vi "test.vi"() -> ()   [LabVIEW 2017]
uses:
  Global/Global 1.vi
panel:
  in  "send":bool
  in  "stop":bool
  in  "scan 6":string
  in  "scan 5":string
  in  "scan 4":string
  in  "scan 3":string
  in  "scan 2":string
  in  "scan 1":string
  in  "cycle start 6":bool
  in  "cycle start 5":bool
  in  "cycle start 4":bool
  in  "cycle start 3":bool
  in  "cycle start 2":bool
  in  "result  6":bool
  in  "cycle start 1":bool
  in  "result  5":bool
  in  "result  4":bool
  in  "result  3":bool
  in  "result  2":bool
  in  "result 1":bool
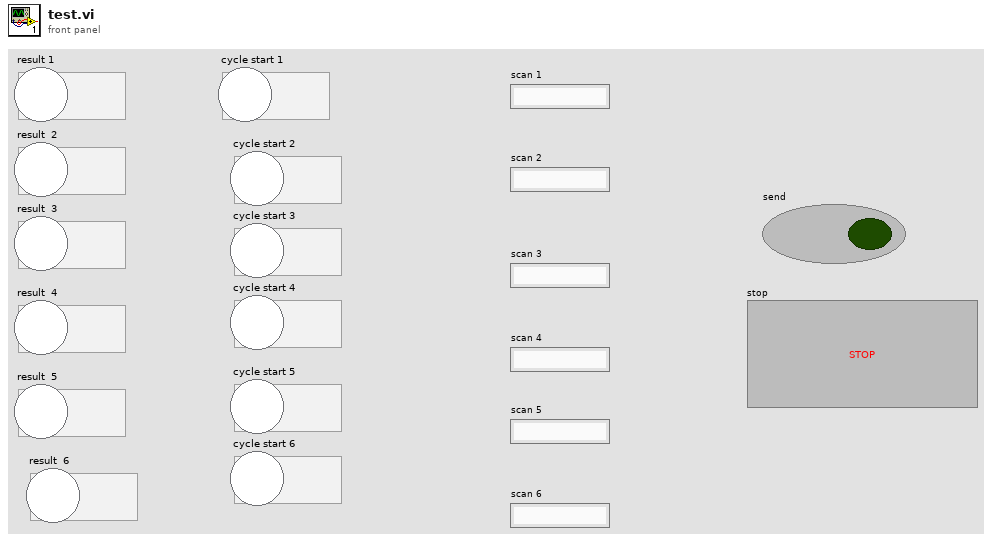
[diagram p1: front panel]
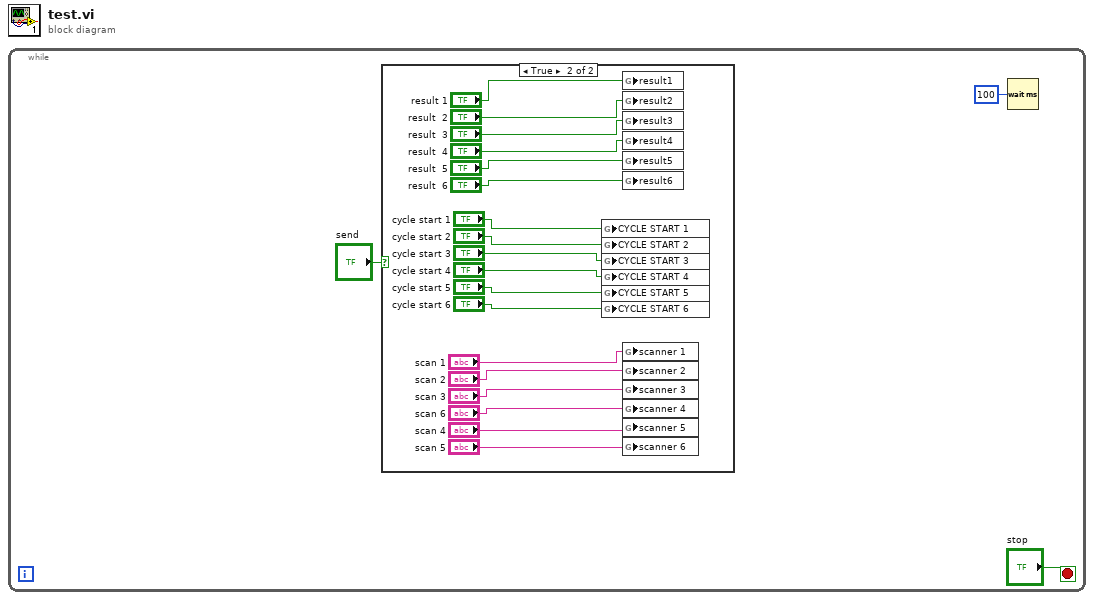
[diagram p0: block diagram]
diagram:
  n1 = while {
    stop <- "stop" stop-if-true
    n2 = case shown="True" "send" {
      frame False {
      }
      frame True {
        n3 = global write "Global 1.vi" "CYCLE START 1"("cycle start 1") -> ()
        n4 = global write "Global 1.vi" "CYCLE START 2"("cycle start 2") -> ()
        n5 = global write "Global 1.vi" "CYCLE START 3"("cycle start 3") -> ()
        n6 = global write "Global 1.vi" "CYCLE START 4"("cycle start 4") -> ()
        n7 = global write "Global 1.vi" "CYCLE START 5"("cycle start 5") -> ()
        n8 = global write "Global 1.vi" "CYCLE START 6"("cycle start 6") -> ()
        n9 = global write "Global 1.vi" "result1"("result 1") -> ()
        n10 = global write "Global 1.vi" "result2"("result  2") -> ()
        n11 = global write "Global 1.vi" "result3"("result  3") -> ()
        n12 = global write "Global 1.vi" "result4"("result  4") -> ()
        n13 = global write "Global 1.vi" "result5"("result  5") -> ()
        n14 = global write "Global 1.vi" "result6"("result  6") -> ()
        n15 = global write "Global 1.vi" "scanner 1"("scan 1") -> ()
        n16 = global write "Global 1.vi" "scanner 2"("scan 2") -> ()
        n17 = global write "Global 1.vi" "scanner 3"("scan 3") -> ()
        n18 = global write "Global 1.vi" "scanner 4"("scan 6") -> ()
        n19 = global write "Global 1.vi" "scanner 5"("scan 4") -> ()
        n20 = global write "Global 1.vi" "scanner 6"("scan 5") -> ()
      }
    }
    n21 = Wait (ms)(milliseconds to wait=u32 100) -> ()  [unwired: 1 out]
  }
